vi "d calc w x.vi"(4 "YP":dbl) -> (0 "d":dbl)   [LabVIEW 2016]
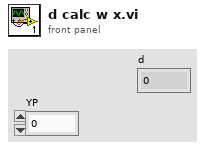
[diagram p1: front panel]
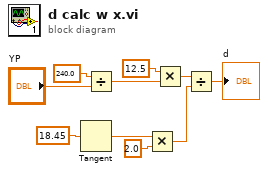
[diagram p0: block diagram]
diagram:
  n1 = Tangent(1:18.45 ("x")) -> (0:w4:dbl)
  n2 = Divide(x=240.0, y="YP") -> (x/y=w9:dbl)
  n3 = Multiply(x=w4, y=2.0) -> (x*y=w2:dbl)
  n4 = Multiply(x=12.5, y=w9) -> (x*y=w7:dbl)
  n5 = Divide(x=w7, y=w2) -> (x/y=→"d":dbl)
